vi "Release Sequence File.vi"(7 "SequenceFile":refnum<k7>, 8 "error in (no error)":errorcluster, 11 "Session Handle in":T1) -> (0 "error out":errorcluster, 3 "Session Handle out":T1)   [LabVIEW 2020, in "TSS.lvlib" / "Engine.lvclass"]
uses:
  Engine/Engine.lvclass
  Engine/Typedefs/Session Handle.ctl
  Engine/Engine.lvclass/Engine.ctl
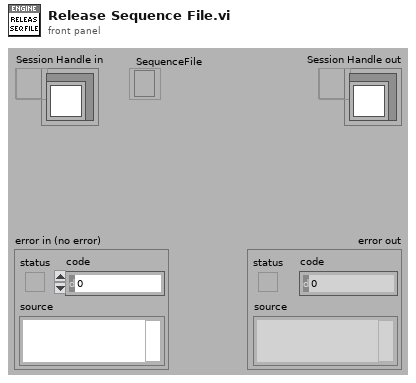
[diagram p1: front panel]
types:
  T1 = typedef "TSS.lvlib/Engine.lvclass/Session Handle.ctl" = refnum<data-value>
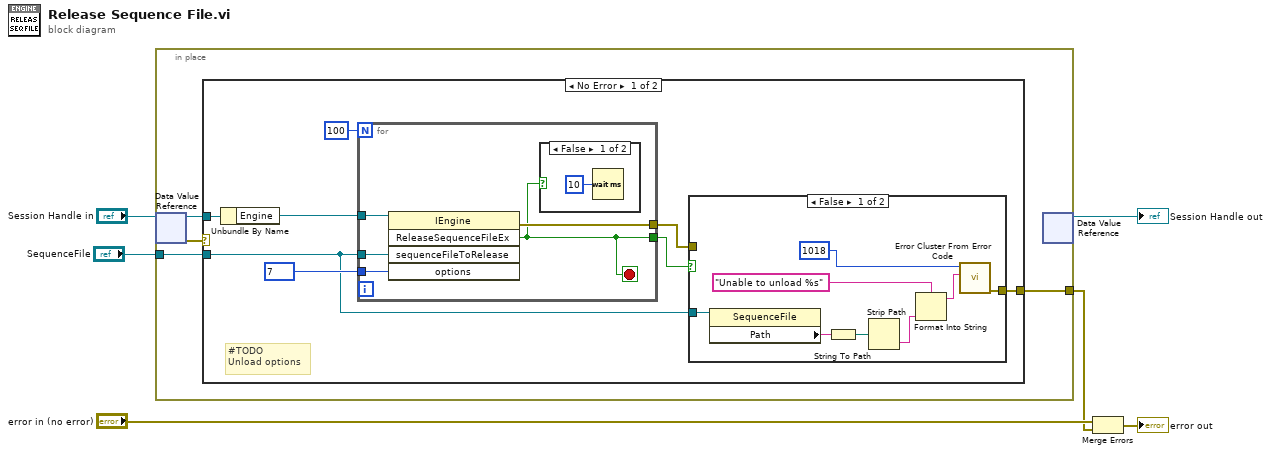
[diagram p0: block diagram]
diagram:
  n1 = in-place {
    in-place-border: "SequenceFile" -> [w8]
    in-place-border: [w7] -> w1
    n2 = in-place-dvr #1("Session Handle in") -> (w9:refnum<class "Engine.lvclass">, w10:errorcluster)
    n3 = case shown="No Error" w10 {
      selector: w10 -> [_ w34]
      tunnel: w9 -> [w18 _]
      tunnel: w8 -> [w11 _]
      tunnel: [w13 w34] -> w7
      frame No Error {
        # "#TODO\nUnload options"
        n4 = Unbundle By Name(w18) -> ("Engine"=w17:refnum<k7>)
        n5 = for {
          N: 100 -> [_]
          tunnel: w17 -> [w23]
          tunnel: w11 -> [w22]
          tunnel: 7 ("options") -> [w21]
          tunnel: [w19] -> w15
          tunnel: [w20] -> w14
          stop <- w19 stop-if-true
          n6 = invoke class="IEngine" method="ReleaseSequenceFileEx"(reference=w23, "sequenceFileToRelease"=w22, "options"=w21) -> (error out=w20:errorcluster, "ReleaseSequenceFileEx"=w19:bool)  [unwired: 2 in, 3 out]
          n7 = case shown="False" w19 {
            frame False {
              n8 = Wait (ms)(milliseconds to wait=u32 10) -> ()  [unwired: 1 out]
            }
            frame True {
            }
          }
        }
        n9 = case shown="False" w15 {
          tunnel: w14 -> [_ w33]
          tunnel: [w31 w33] -> w13
          tunnel: w11 -> [w30 _]
          frame False {
            n10 = property class="SequenceFile"(reference=w30) -> ("Path"=w29:string)  [unwired: 1 in, 2 out]
            n11 = String To Path(string=w29) -> (path=w28:path)
            n12 = Strip Path(path=w28) -> (name=w26:string)  [unwired: 1 out]
            n13 = Format Into String(format string="Unable to unload %s" ("error message (\"\")"), w26) -> (resulting string=w25:string)  [unwired: 2 in, 1 out]
            n14 = call <vilib>:"Error Cluster From Error Code.vi"("error message (\"\")"=w25, "error code (0)"=1018) -> ("error out"=w31:errorcluster)  [unwired: 7 in]
          }
          frame True {
          }
        }
      }
      frame Error {
      }
    }
    n15 = in-place-dvr #1() -> (→"Session Handle out":T1)  [unwired: 1 in, 1 out]
  }
  n16 = Merge Errors("error in (no error)", w1) -> (→"error out":errorcluster)
